vi "Wait for First Request.vi"(8 "error in (no error)":errorcluster, 11 "Elevator Controller in":refnum<class "Elevator Controller.lvclass">) -> (0 "error out":errorcluster, 3 "Elevator Controller out":refnum<class "Elevator Controller.lvclass">)   [LabVIEW 2019, in "Elevator Controller.lvlib" / "Elevator Controller.lvclass"]
uses:
  Elevator Controller.lvclass
  State -Enum.ctl
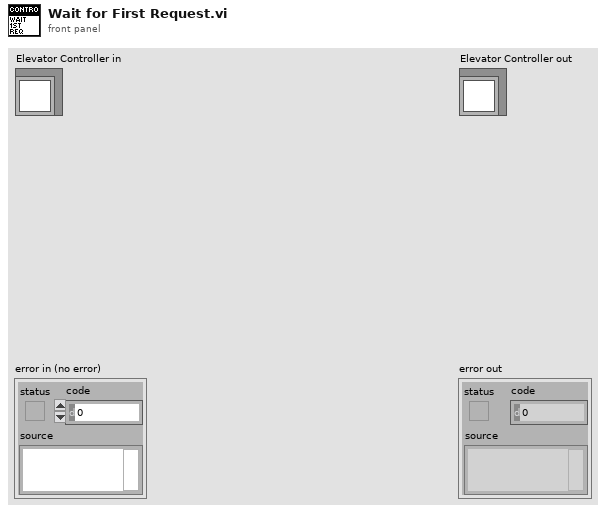
[diagram p1: front panel]
types:
  T1 = typedef "Elevator Controller.lvlib/Elevator Controller.lvclass/State -Enum.ctl" = enum16{"Initial", "Wait for First Request", "Start and Move", "Analysis", "Continue Travel", "Stop at Floor", "Open and Close Door Sequence", "No request Remaining", "Emergency Call", "Terminate Process"}
  T2 = typedef "Sim Display Console Actor.lvlib/Sim Display Console Actor.lvclass/Floors -Enum.ctl" = enum16{"1st Floor", "2nd Floor", "3rd Floor", "4th Floor"}
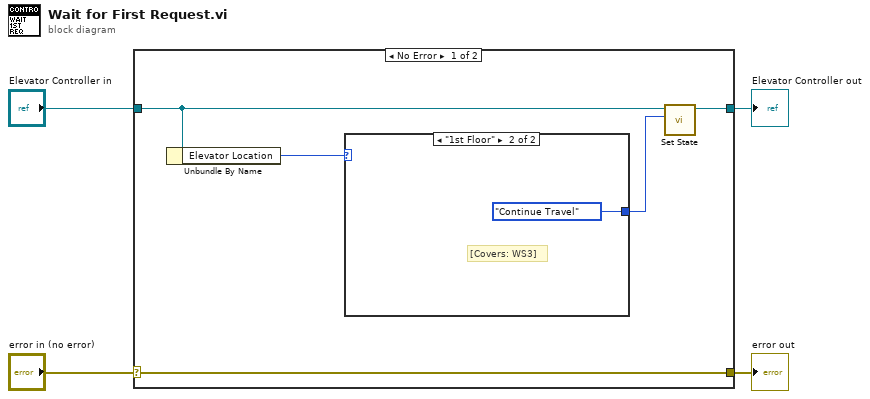
[diagram p0: block diagram]
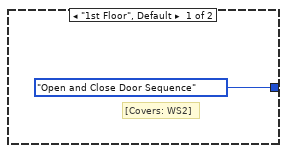
[diagram p2: hidden frame]
diagram:
  n1 = case shown="No Error" "error in (no error)" {
    selector: "error in (no error)" -> [w9 w13]
    tunnel: [w9 w13] -> w3
    tunnel: [w6 w12] -> w1
    tunnel: "Elevator Controller in" -> [w7 w12]
    frame No Error {
      n2 = Unbundle By Name(w7) -> ("Elevator Location"=w8:T2)
      n3 = case shown="\"Anathor Floors\"" w8 {
        tunnel: [State_-Enum."Open and Close Door Sequence" ("State") State_-Enum."Continue Travel" ("State")] -> w5
        frame "1st Floor", Default {
          # "[Covers: WS2]"
        }
        frame "1st Floor" {
          # "[Covers: WS3]"
        }
      }
      n4 = call "Set State.vi"("State"=w5, "Elevator Controller in"=w7) -> ("Elevator Controller out"=w6:refnum<class "Elevator Controller.lvclass">)  [unwired: 8 in, 1 out]
    }
    frame Error {
    }
  }
  "error out" <- w3
  "Elevator Controller out" <- w1
